vi "qc5psm3.vi"() -> ()   [LabVIEW 2020]
uses:
  <instrlib>/CAEN PSM/CAEN PSM.lvlib
panel:
  in  "Tab Control":enum32{"Page 1"}(tab)
  in  "Tab Control 3":enum32{"Page 1", "Page 2", "Page 3"}(tab)
  out "XY Graph":cluster{"X":dbl, "Y":dbl}[](graph)
  out "XY Graph 2":cluster{"X":dbl, "Y":dbl}[](graph)
  out "XY Graph 3":cluster{"Y":dbl[], "Y":dbl[]}[](graph)
  out "STATUS":string
  in  "Tab Control 2":enum32{"Page 1", "Page 2"}(tab)
  out "RDW":bool
  out "VMON":dbl(graph)
  out "IMON":dbl(graph)
  out "Shutting  DOWN":bool
  out "Vmon (Actual voltage level )":dbl
  out "Imon (Actual current level )":dbl
  out "OVC 2":bool
  out "OVV 2":bool
  out "COUNT VALUE":dynamicdata(graph)
  in  "count Time(sec)":dbl=60.0
  in  "Final Voltage":dbl=4900.0
  in  "V_step 1":dbl=200.0
  in  "VISA resource name":refnum<visa-resource-name>
  in  "Voltage ramp up (0 V/s)":u16 max=999
  in  "Voltage Max (0.0 V)":u16 max=9999
  in  "Board Address":i8 max=31
  in  "Vset_initial":dbl=200.0
  out "R calc":dbl
  in  "START AGAIN":bool
  out "Channel Status":T1(array[cluster])
  in  "Channel (0)":u8=1
  in  "Req (Mohm)":dbl
  in  "stop":bool
  in  "Middle Volt":dbl=3000.0
  in  "V step 2":dbl=100.0
  out "COUNT ON  TIMES":i16
  in  "device name (NI USB 6009)":tag="Dev1"
  out "Counts":dbl
  out "time eclapsed":i32
  out "I set status":dbl
  # "VOLTAGE RAMPUP SCHEME"
  # "INITIAL SETTING"
  # "RATE MEASUREMENT"
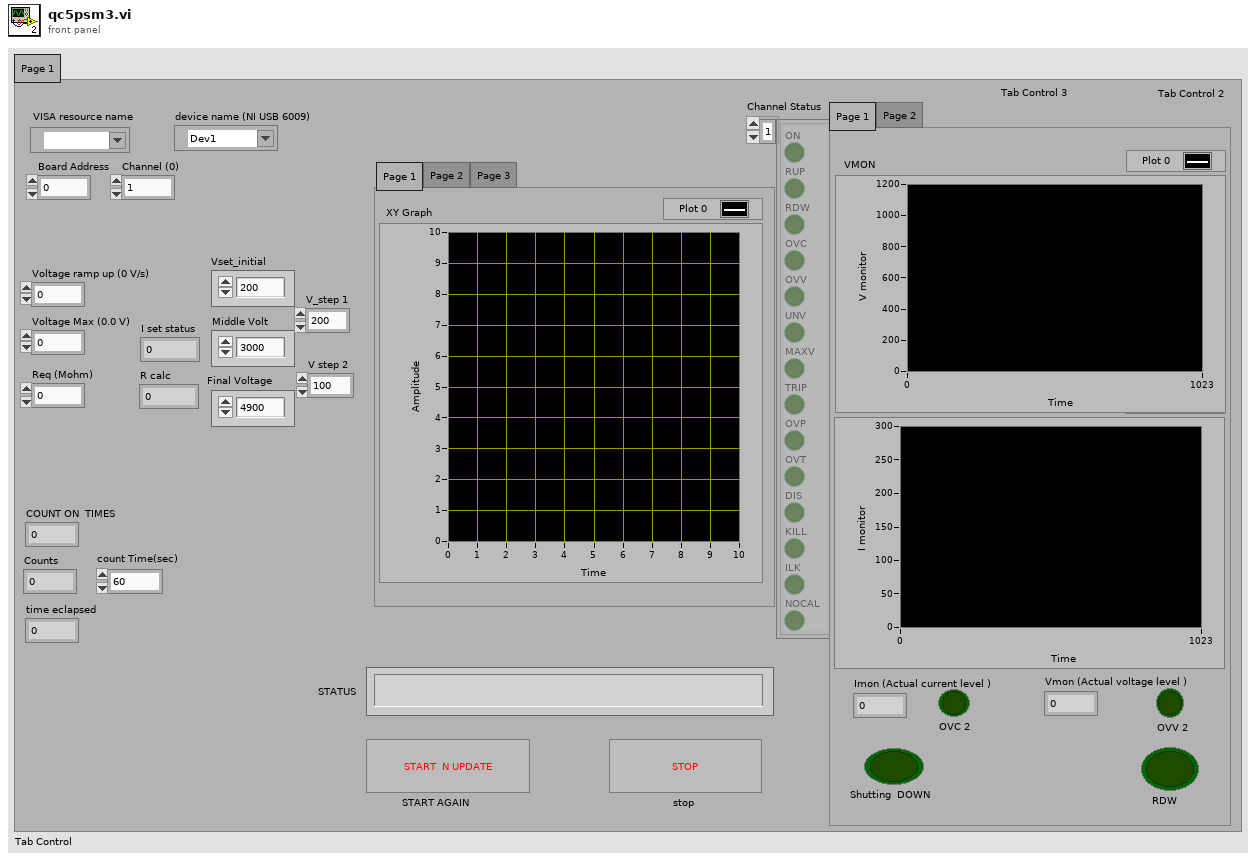
[diagram p1: front panel]
types:
  T1 = cluster{"ON":bool, "RUP":bool, "RDW":bool, "OVC":bool, "OVV":bool, "UNV":bool, "MAXV":bool, "TRIP":bool, "OVP":bool, "OVT":bool, "DIS":bool, "KILL":bool, "ILK":bool, "NOCAL":bool}[]
  T2 = cluster{"Baud Rate":u32, "Parity":enum16{"None", "Odd", "Even", "Mark", "Space"}, "Data Bits":u16, "Stop Bits":u16, "Flow Control":u16}
  T3 = typedef "CAEN PSM.lvlib/BoardHandle.ctl" = cluster{"VISA resource name":refnum<visa-resource-name>, "Board address":i8, "NChannels":u8}
  T4 = cluster{"ON":bool, "RUP":bool, "RDW":bool, "OVC":bool, "OVV":bool, "UNV":bool, "MAXV":bool, "TRIP":bool, "OVP":bool, "OVT":bool, "DIS":bool, "KILL":bool, "ILK":bool, "NOCAL":bool}
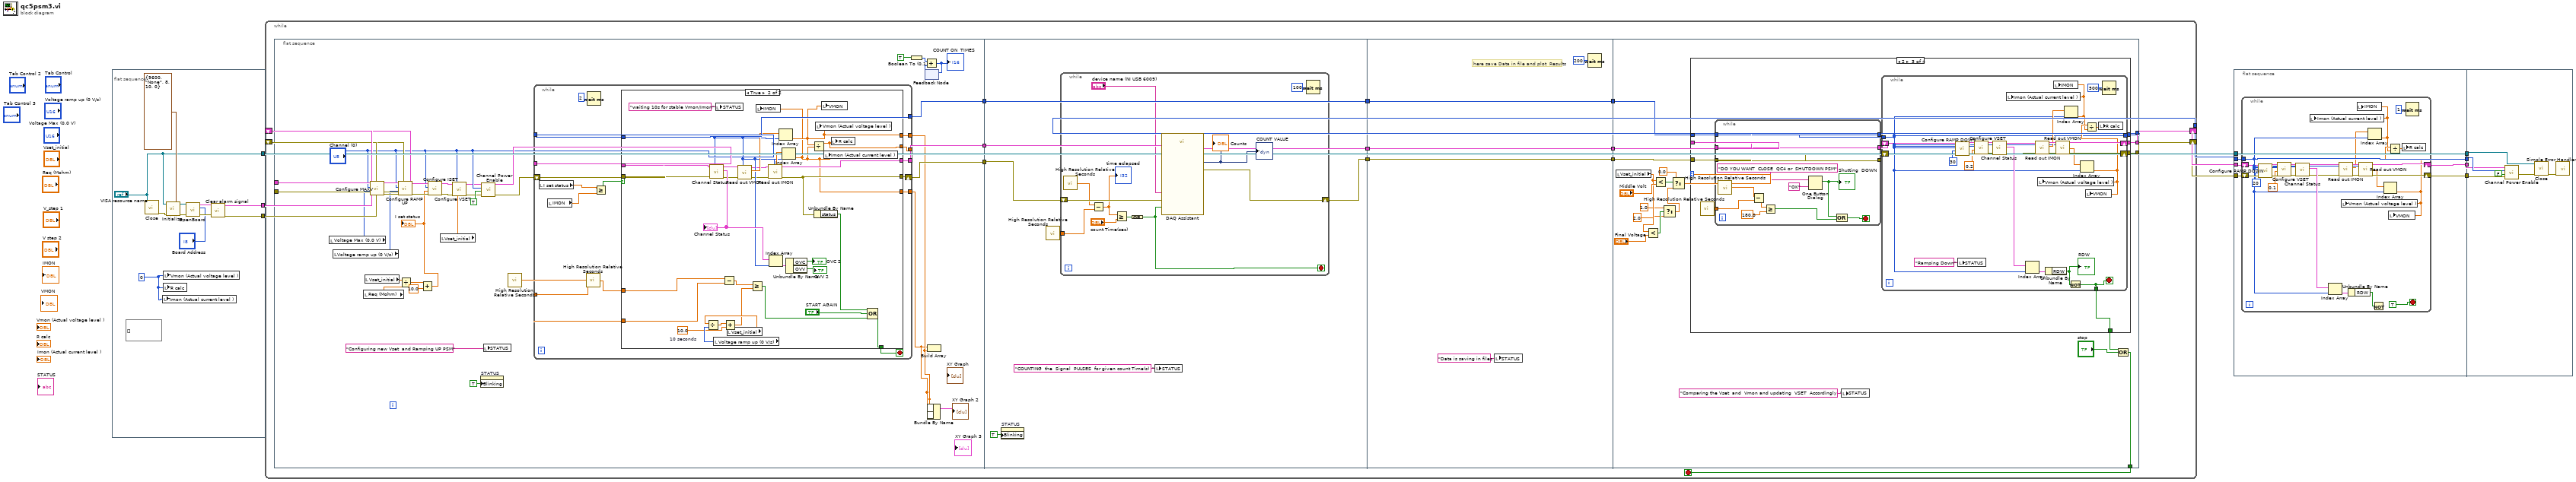
[diagram p0: block diagram]
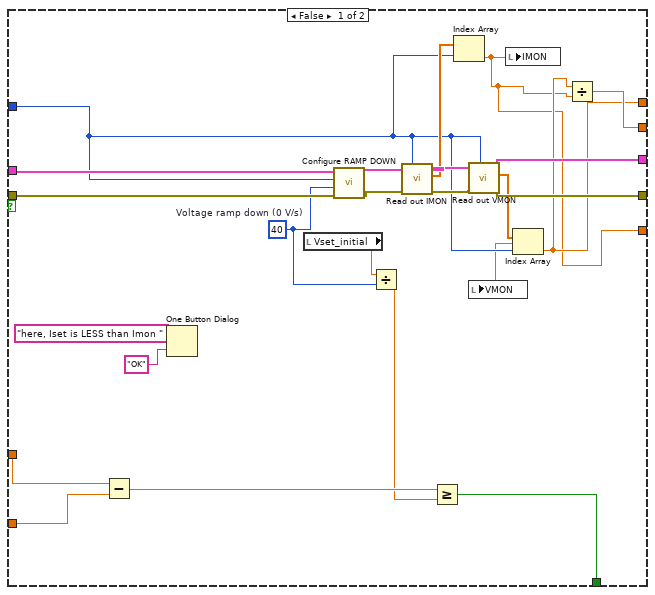
[diagram p2: hidden frame]
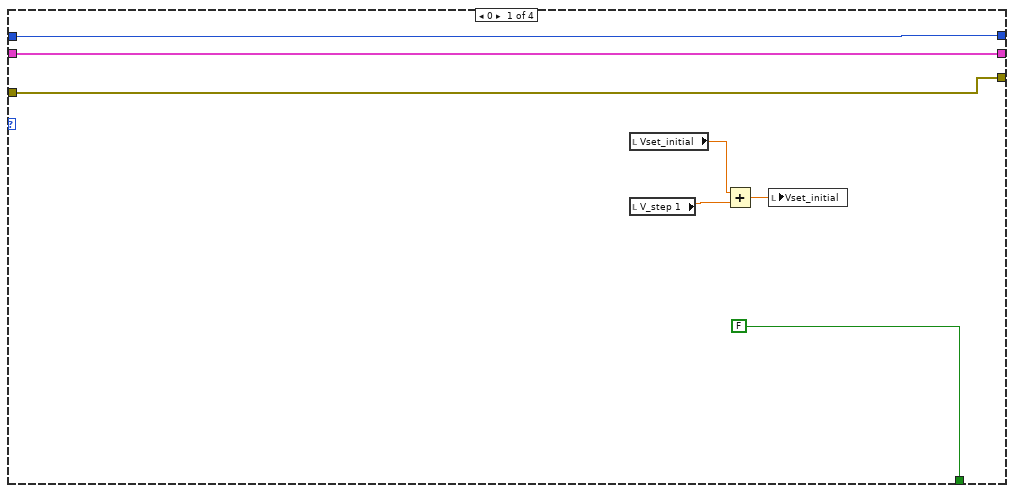
[diagram p3: hidden frame]
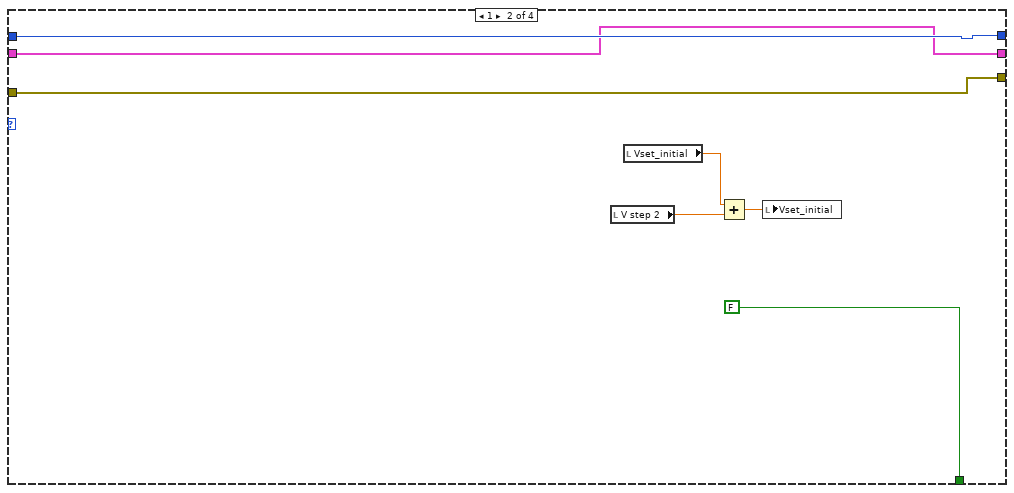
[diagram p4: hidden frame]
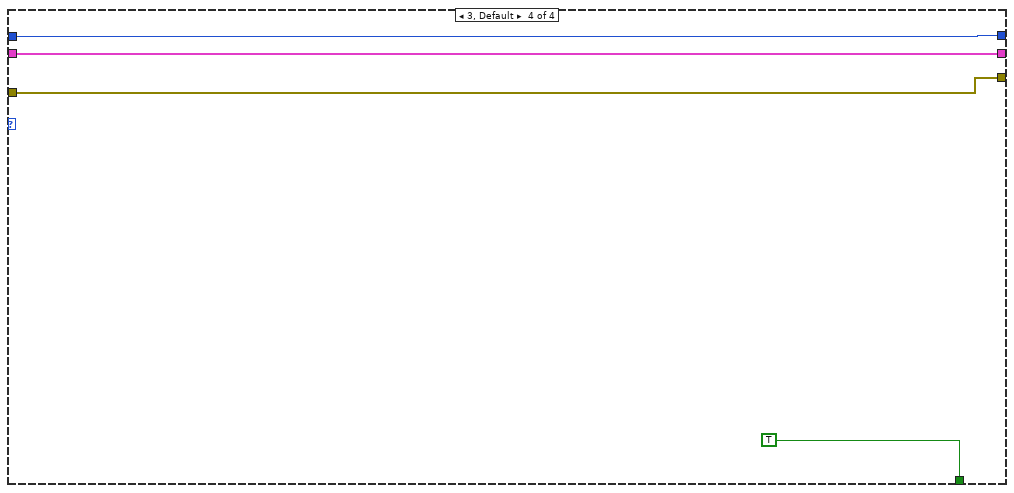
[diagram p5: hidden frame]
diagram:
  n1 = flat-sequence {
    tunnel: ["VISA resource name"] -> w10
    tunnel: [w15] -> w8
    tunnel: [w14] -> w7
    frame #0 {
      (unwired) void[][] []
      w11 = 0
      n2 = call <instrlib>:"Close.vi"("VISA resource name"="VISA resource name") -> ("error out"=w13:errorcluster)  [unwired: 10 in]
      n3 = local write "Imon (Actual current level )"(w11) -> ()
      n4 = local write "Vmon (Actual voltage level )"(w11) -> ()
      n5 = local write "R calc"(w11) -> ()
      n6 = call <instrlib>:"Initialize.vi"("Serial Configuration"=T2 {"Baud Rate"=9600, "Parity"=enum."None", "Data Bits"=8, "Stop Bits"=10, "Flow Control"=0}, "error in (no error)"=w13, "VISA resource name"="VISA resource name") -> ("error out"=w12:errorcluster, "VISA resource name out"=w20:refnum<visa-resource-name>)  [unwired: 7 in]
      n7 = call <instrlib>:"OpenBoard.vi"("error in (no error)"=w12, "Board Address"="Board Address", "VISA resource name"=w20) -> ("error out"=w18:errorcluster, "BoardHandle"=w19:T3)  [unwired: 7 in]
      n8 = call <instrlib>:"Clear alarm signal.vi"("error in (no error)"=w18, "BoardHandle"=w19) -> ("error out"=w14:errorcluster, "BoardHandle out"=w15:T3)  [unwired: 8 in]
    }
  }
  n9 = while {
    tunnel: [w36] -> w9
    shift-right: [w33] -> w6
    shift-left: w8 -> [w35]
    shift-right: [w28] -> w5
    shift-left: w7 -> [w34]
    stop <- w32 stop-if-true
    n10 = flat-sequence {
      tunnel: [w73] -> w31
      tunnel: [w52] -> w30
      tunnel: [w51] -> w29
      tunnel: w35 -> [w72]
      tunnel: w34 -> [w71]
      tunnel: w31 -> [w150]
      tunnel: [w150] -> w27
      tunnel: w30 -> [w149]
      tunnel: [w149] -> w25
      tunnel: w29 -> [w148]
      tunnel: [w147] -> w23
      tunnel: w27 -> [w166]
      tunnel: [w166] -> w26
      tunnel: w25 -> [w165]
      tunnel: [w165] -> w24
      tunnel: w23 -> [w164]
      tunnel: [w164] -> w22
      tunnel: [w169] -> w28
      tunnel: [w168] -> w33
      tunnel: [w172] -> w36
      tunnel: w26 -> [w173]
      tunnel: w24 -> [w171]
      tunnel: w22 -> [w170]
      tunnel: [w175] -> w32
      frame #0 {
        n11 = local read "Voltage Max (0.0 V)"() -> (w67:u16)
        n12 = local read "Voltage ramp up (0 V/s)"() -> (w66:u16)
        n13 = local read "Req (Mohm)"() -> (w56:dbl)
        n14 = local read "Vset_initial"() -> (w57:dbl)
        n15 = call <instrlib>:"Configure MAXV.vi"("error in (no error)"=w71, "Voltage Max (0.0 V)"=w67, "Channel (0)"="Channel (0)", "BoardHandle"=w72) -> ("error out"=w68:errorcluster, "BoardHandle out"=w69:T3)  [unwired: 6 in]
        n16 = call <instrlib>:"Configure RAMP UP.vi"("error in (no error)"=w68, "Voltage ramp up (0 V/s)"=w66, "Channel (0)"="Channel (0)", "BoardHandle"=w69) -> ("error out"=w62:errorcluster, "BoardHandle out"=w64:T3)  [unwired: 6 in]
        n17 = Divide(x=w57, y=w56) -> (x/y=w59:dbl)
        n18 = Add(x=w59, y=10.0) -> (x+y=w49:dbl)
        "I set status" <- w49
        n19 = call <instrlib>:"Configure ISET.vi"("error in (no error)"=w62, "Current Limit (0.00 uA)"=w49, "Channel (0)"="Channel (0)", "BoardHandle"=w64) -> ("error out"=w61:errorcluster, "BoardHandle out"=w63:T3)  [unwired: 6 in]
        n20 = local read "Vset_initial"() -> (w60:dbl)
        n21 = call <instrlib>:"Configure VSET.vi"("error in (no error)"=w61, "Voltage Level (0.0 V)"=w60, "Channel (0)"="Channel (0)", "BoardHandle"=w63) -> ("error out"=w54:errorcluster, "BoardHandle out"=w53:T3)  [unwired: 6 in]
        n22 = property on="STATUS" class="Str"("Blinking"=TRUE) -> ()  [unwired: 2 in, 2 out]
        n23 = call <instrlib>:"Channel Power Enable.vi"("error in (no error)"=w54, "Enable (OFF)"=TRUE, "Channel (0)"="Channel (0)", "BoardHandle"=w53) -> ("error out"=w70:errorcluster, "BoardHandle out"=w74:T3)  [unwired: 6 in]
        n24 = local write "STATUS"("Configuring new Vset  and Ramping UP PSM" ("STATUS")) -> ()
        n25 = call <vilib>:"High Resolution Relative Seconds.vi"() -> ("relative seconds"=w50:dbl)
        n26 = while {
          shift-right: [w85] -> w51
          shift-left: w70 -> [w86]
          tunnel: [w84] -> w52
          tunnel: [w89] -> w73
          tunnel: w74 -> [w87]
          tunnel: "Channel (0)" -> [w89]
          tunnel: w50 -> [w82]
          tunnel: [w77] -> w38
          tunnel: [w75] -> w42
          tunnel: [w76] -> w37
          stop <- w81 stop-if-true
          n27 = local read "I set status"() -> (w80:dbl)
          n28 = local read "IMON"() -> (w78:dbl)
          n29 = call <vilib>:"High Resolution Relative Seconds.vi"() -> ("relative seconds"=w79:dbl)
          n30 = Wait (ms)(milliseconds to wait=u32 2) -> ()  [unwired: 1 out]
          n31 = Greater Or Equal?(x=w80, y=w78) -> (x >= y?=w83:bool)
          n32 = case shown="True" w83 {
            tunnel: w89 -> [w96 w137]
            tunnel: w87 -> [w112 w136]
            tunnel: w86 -> [w111 w135]
            tunnel: [w99 w134] -> w85
            tunnel: [w100 w133] -> w84
            tunnel: w82 -> [w110 w128]
            tunnel: [w105 w123] -> w81
            tunnel: w79 -> [w93 w117]
            tunnel: [w91 w115] -> w77
            tunnel: [w90 w114] -> w76
            tunnel: [w92 w113] -> w75
            frame False {
              w107 = u16 40  # Voltage ramp down (0 V/s)
              n33 = Subtract(x=w93, y=w110) -> (x-y=w109:dbl)
              n34 = One Button Dialog(message="here, Iset is LESS than Imon ", button name ("OK")="OK") -> ()  [unwired: 1 out]
              n35 = local read "Vset_initial"() -> (w108:dbl)
              n36 = call <instrlib>:"Configure RAMP DOWN.vi"("error in (no error)"=w111, "Voltage ramp down (0 V/s)"=w107, "Channel (0)"=w96, "BoardHandle"=w112) -> ("error out"=w103:errorcluster, "BoardHandle out"=w104:T3)  [unwired: 6 in]
              n37 = Divide(x=w108, y=w107) -> (x/y=w106:dbl)
              n38 = call <instrlib>:"Read out IMON.vi"("Channel"=w96, "error in (no error)"=w103, "BoardHandle"=w104) -> ("error out"=w101:errorcluster, "IMon values (uA)"=w98:dbl[], "BoardHandle out"=w102:T3)  [unwired: 5 in, 1 out]
              n39 = Greater Or Equal?(x=w109, y=w106) -> (x >= y?=w105:bool)
              n40 = Index Array(array=w98, index=w96) -> (element=w90:dbl)
              n41 = call <instrlib>:"Read out VMON.vi"("Channel"=w96, "error in (no error)"=w101, "BoardHandle"=w102) -> ("error out"=w99:errorcluster, "VMon values (V)"=w97:dbl[], "BoardHandle out"=w100:T3)  [unwired: 6 in]
              n42 = local write "IMON"(w90) -> ()
              n43 = Index Array(array=w97, index=w96) -> (element=w91:dbl)
              n44 = local write "VMON"(w91) -> ()
              n45 = Divide(x=w91, y=w90) -> (x/y=w92:dbl)
            }
            frame True {
              w119 = 10.0  # 10 seconds
              n46 = call <instrlib>:"Channel Status.vi"("Channel"=w137, "error in (no error)"=w135, "BoardHandle"=w136) -> ("error out"=w131:errorcluster, "Channel Status Array"=w142:T1, "BoardHandle out"=w132:T3)  [unwired: 5 in, 1 out]
              "Channel Status" <- w142
              n47 = local read "Voltage ramp up (0 V/s)"() -> (w121:u16)
              n48 = local write "STATUS"("waiting 10s for stable Vmon/Imon" ("STATUS")) -> ()
              n49 = Subtract(x=w117, y=w128) -> (x-y=w125:dbl)
              n50 = local read "Vset_initial"() -> (w122:dbl)
              n51 = Divide(x=w122, y=w121) -> (x/y=w120:dbl)
              n52 = Add(x=w120, y=w119) -> (x+y=w118:dbl)
              n53 = call <instrlib>:"Read out VMON.vi"("Channel"=w137, "error in (no error)"=w131, "BoardHandle"=w132) -> ("error out"=w129:errorcluster, "VMon values (V)"=w143:dbl[], "BoardHandle out"=w130:T3)  [unwired: 6 in]
              n54 = Greater Or Equal?(x=w125, y=w118) -> (x >= y?=w127:bool)
              n55 = call <instrlib>:"Read out IMON.vi"("Channel"=w137, "error in (no error)"=w129, "BoardHandle"=w130) -> ("error out"=w134:errorcluster, "IMon values (uA)"=w138:dbl[], "BoardHandle out"=w133:T3)  [unwired: 5 in, 1 out]
              n56 = Index Array(array=w142, index=w137) -> (element=w141:T4)
              n57 = Index Array(array=w143, index=w137) -> (element=w115:dbl)
              n58 = Index Array(array=w138, index=w137) -> (element=w114:dbl)
              n59 = local write "IMON"(w114) -> ()
              n60 = Unbundle By Name(w141) -> ("OVC"=→"OVC 2":bool, "OVV"=→"OVV 2":bool)
              n61 = Divide(x=w115, y=w114) -> (x/y=w113:dbl)
              n62 = Unbundle By Name(w134) -> ("status"=w124:bool)
              n63 = local write "Vmon (Actual voltage level )"(w115) -> ()
              n64 = local write "VMON"(w115) -> ()
              n65 = local write "Imon (Actual current level )"(w114) -> ()
              n66 = local write "R calc"(w113) -> ()
              n67 = Compound Arithmetic op=OR(w124, "START AGAIN", w127) -> (w123:bool)
            }
          }
        }
        n68 = Boolean To (0,1)(Boolean=TRUE) -> (0, 1=w46:i16)
        n69 = feedback #1() -> (w48:i16)  [unwired: 1 in]
        n70 = Add(x=w46, y=w48) -> (x+y=w47:i16)
        "COUNT ON  TIMES" <- w47
        n71 = feedback-in #1(w47) -> ()
        n72 = Build Array(w37, w38) -> (w40:dbl[])
        n73 = Bundle By Name(w38, w37) -> (→"XY Graph 2":cluster{})  [unwired: 1 in]
      }
      frame #1 {
        n74 = property on="STATUS" class="Str"("Blinking"=TRUE) -> ()  [unwired: 2 in, 2 out]
        n75 = call <vilib>:"High Resolution Relative Seconds.vi"() -> ("relative seconds"=w146:dbl)
        n76 = while {
          shift-right: [w160] -> w147
          shift-left: w148 -> [w161]
          tunnel: w146 -> [w155]
          stop <- w152 stop-if-true
          n77 = call <vilib>:"High Resolution Relative Seconds.vi"() -> ("relative seconds"=w157:dbl)
          n78 = Subtract(x=w157, y=w155) -> (x-y=w158:dbl)
          "time eclapsed" <- w158
          n79 = Greater Or Equal?(x=w158, y="count Time(sec)") -> (x >= y?=w156:bool)
          n80 = Compound Arithmetic op=OR(w156) -> (w152:bool)
          n81 = call "DAQ Assistant"("error in"=w161, "stop (F)"=w152, "device name"="device name (NI USB 6009)") -> ("data"=→"Counts" →"COUNT VALUE":dynamicdata, "error out"=w160:errorcluster)  [unwired: 13 in, 2 out]
          n82 = Wait (ms)(milliseconds to wait=u32 100) -> ()  [unwired: 1 out]
        }
        n83 = local write "STATUS"("COUNTING  the  Signal  PULSES  for given count Time(s)  " ("STATUS")) -> ()
      }
      frame #2 {
        # "here save Data in file and plot  Results"
        n84 = local write "STATUS"("Data is saving in files " ("STATUS")) -> ()
        n85 = Wait (ms)(milliseconds to wait=u32 200) -> ()  [unwired: 1 out]
      }
      frame #3 {
        n86 = local read "Vset_initial"() -> (w180:dbl)
        n87 = Less?(x=w180, y="Final Voltage") -> (x < y?=w183:bool)
        n88 = Less?(x=w180, y="Middle Volt") -> (x < y?=w185:bool)
        n89 = Select(t=1.0, s=w183, f=2.0) -> (s? t:f=w181:dbl)
        n90 = Select(t=0.0, s=w185, f=w181) -> (s? t:f=w186:dbl)
        n91 = case shown="2" w186 {
          tunnel: [FALSE FALSE w208 TRUE] -> w174
          tunnel: w173 -> [w189 w196 w203 w251]
          tunnel: [w189 w196 w211 w251] -> w172
          tunnel: w171 -> [w188 w195 w205 w250]
          tunnel: w170 -> [w187 w194 w207 w249]
          tunnel: [w187 w194 w209 w249] -> w169
          tunnel: [w188 w195 w210 w250] -> w168
          frame 0 {
            n92 = local read "Vset_initial"() -> (w193:dbl)
            n93 = local read "V_step 1"() -> (w191:dbl)
            n94 = Add(x=w193, y=w191) -> (x+y=w192:dbl)
            n95 = local write "Vset_initial"(w192) -> ()
          }
          frame 1 {
            n96 = local read "V step 2"() -> (w198:dbl)
            n97 = local read "Vset_initial"() -> (w200:dbl)
            n98 = Add(x=w200, y=w198) -> (x+y=w199:dbl)
            n99 = local write "Vset_initial"(w199) -> ()
          }
          frame 2 {
            n100 = call <vilib>:"High Resolution Relative Seconds.vi"() -> ("relative seconds"=w201:dbl)
            n101 = while {
              tunnel: w207 -> [w223]
              tunnel: [w223] -> w206
              tunnel: w205 -> [w222]
              tunnel: [w222] -> w204
              tunnel: w203 -> [w221]
              tunnel: [w221] -> w202
              tunnel: w201 -> [w217]
              stop <- w213 stop-if-true
              n102 = call <vilib>:"High Resolution Relative Seconds.vi"() -> ("relative seconds"=w218:dbl)
              n103 = Subtract(x=w218, y=w217) -> (x-y=w216:dbl)
              n104 = Greater Or Equal?(x=w216, y=180.0) -> (x >= y?=w214:bool)
              n105 = One Button Dialog(message="DO YOU WANT  CLOSE  QC4 or  SHUTDOWN PSM", button name ("OK")="OK") -> (true=w212:bool)
              "Shutting  DOWN" <- w212
              n106 = Compound Arithmetic op=OR(w212, w214) -> (w213:bool)
            }
            n107 = while {
              tunnel: w202 -> [w226]
              shift-right: [w246] -> w210
              shift-left: w204 -> [w248]
              shift-right: [w245] -> w209
              shift-left: w206 -> [w247]
              tunnel: [w226] -> w211
              tunnel: [w225] -> w208
              stop <- w225 stop-if-true
              n108 = call <instrlib>:"Configure RAMP DOWN.vi"("error in (no error)"=w247, "Voltage ramp down (0 V/s)"=u16 30, "Channel (0)"=w226, "BoardHandle"=w248) -> ("error out"=w241:errorcluster, "BoardHandle out"=w242:T3)  [unwired: 6 in]
              n109 = local write "STATUS"("Ramping Down" ("STATUS")) -> ()
              n110 = call <instrlib>:"Configure VSET.vi"("error in (no error)"=w241, "Voltage Level (0.0 V)"=0.2, "Channel (0)"=w226, "BoardHandle"=w242) -> ("error out"=w238:errorcluster, "BoardHandle out"=w239:T3)  [unwired: 6 in]
              n111 = call <instrlib>:"Channel Status.vi"("Channel"=w226, "error in (no error)"=w238, "BoardHandle"=w239) -> ("error out"=w233:errorcluster, "Channel Status Array"=w237:T1, "BoardHandle out"=w232:T3)  [unwired: 5 in, 1 out]
              n112 = Index Array(array=w237, index=w226) -> (element=w236:T4)
              n113 = call <instrlib>:"Read out IMON.vi"("Channel"=w226, "BoardHandle"=w232) -> ("IMon values (uA)"=w230:dbl[], "BoardHandle out"=w231:T3)  [unwired: 6 in, 2 out]
              n114 = Unbundle By Name(w236) -> ("RDW"=w235:bool)
              "RDW" <- w235
              n115 = call <instrlib>:"Read out VMON.vi"("Channel"=w226, "error in (no error)"=w233, "BoardHandle"=w231) -> ("error out"=w245:errorcluster, "VMon values (V)"=w243:dbl[], "BoardHandle out"=w246:T3)  [unwired: 6 in]
              n116 = Index Array(array=w230, index=w226) -> (element=w227:dbl)
              n117 = local write "Imon (Actual current level )"(w227) -> ()
              n118 = local write "IMON"(w227) -> ()
              n119 = Not(x=w235) -> (.not. x?=w225:bool)
              n120 = Index Array(array=w243, index=w226) -> (element=w228:dbl)
              n121 = local write "Vmon (Actual voltage level )"(w228) -> ()
              n122 = Divide(x=w228, y=w227) -> (x/y=w229:dbl)
              n123 = local write "VMON"(w228) -> ()
              n124 = local write "R calc"(w229) -> ()
              n125 = Wait (ms)(milliseconds to wait=u32 500) -> ()  [unwired: 1 out]
            }
          }
          frame 3, Default {
          }
        }
        n126 = local write "STATUS"("Comparing the Vset  and  Vmon and updating  VSET  Accordingly  " ("STATUS")) -> ()
        n127 = Compound Arithmetic op=OR(w174, "stop") -> (w175:bool)
      }
    }
  }
  n128 = flat-sequence {
    tunnel: w5 -> [w256]
    tunnel: w6 -> [w257]
    tunnel: w9 -> [w253]
    tunnel: w10 -> [w258]
    tunnel: [w258] -> w4
    tunnel: [w253] -> w3
    tunnel: [w255] -> w2
    tunnel: [w254] -> w1
    tunnel: w4 -> [w287]
    tunnel: w3 -> [w285]
    tunnel: w2 -> [w284]
    tunnel: w1 -> [w283]
    frame #0 {
      n129 = while {
        tunnel: w253 -> [w270]
        shift-right: [w280] -> w255
        shift-left: w257 -> [w282]
        shift-right: [w279] -> w254
        shift-left: w256 -> [w281]
        stop <- TRUE stop-if-true
        n130 = call <instrlib>:"Configure RAMP DOWN.vi"("error in (no error)"=w281, "Voltage ramp down (0 V/s)"=u16 20, "Channel (0)"=w270, "BoardHandle"=w282) -> ("error out"=w275:errorcluster, "BoardHandle out"=w276:T3)  [unwired: 6 in]
        n131 = call <instrlib>:"Configure VSET.vi"("error in (no error)"=w275, "Voltage Level (0.0 V)"=0.1, "Channel (0)"=w270, "BoardHandle"=w276) -> ("error out"=w272:errorcluster, "BoardHandle out"=w273:T3)  [unwired: 6 in]
        n132 = call <instrlib>:"Channel Status.vi"("Channel"=w270, "error in (no error)"=w272, "BoardHandle"=w273) -> ("error out"=w266:errorcluster, "Channel Status Array"=w271:T1, "BoardHandle out"=w265:T3)  [unwired: 5 in, 1 out]
        n133 = Index Array(array=w271, index=w270) -> (element=w269:T4)
        n134 = call <instrlib>:"Read out IMON.vi"("Channel"=w270, "BoardHandle"=w265) -> ("IMon values (uA)"=w263:dbl[], "BoardHandle out"=w264:T3)  [unwired: 6 in, 2 out]
        n135 = Unbundle By Name(w269) -> ("RDW"=w268:bool)
        n136 = call <instrlib>:"Read out VMON.vi"("Channel"=w270, "error in (no error)"=w266, "BoardHandle"=w264) -> ("error out"=w279:errorcluster, "VMon values (V)"=w277:dbl[], "BoardHandle out"=w280:T3)  [unwired: 6 in]
        n137 = Index Array(array=w263, index=w270) -> (element=w260:dbl)
        n138 = local write "Imon (Actual current level )"(w260) -> ()
        n139 = local write "IMON"(w260) -> ()
        n140 = Not(x=w268) -> ()  [unwired: 1 out]
        n141 = Index Array(array=w277, index=w270) -> (element=w261:dbl)
        n142 = local write "Vmon (Actual voltage level )"(w261) -> ()
        n143 = Divide(x=w261, y=w260) -> (x/y=w262:dbl)
        n144 = local write "VMON"(w261) -> ()
        n145 = local write "R calc"(w262) -> ()
        n146 = Wait (ms)(milliseconds to wait=u32 1) -> ()  [unwired: 1 out]
      }
    }
    frame #1 {
      n147 = call <instrlib>:"Channel Power Enable.vi"("error in (no error)"=w283, "Enable (OFF)"=FALSE, "Channel (0)"=w285, "BoardHandle"=w284) -> ("error out"=w289:errorcluster)  [unwired: 6 in, 1 out]
      n148 = call <instrlib>:"Close.vi"("error in (no error)"=w289, "VISA resource name"=w287) -> ("error out"=w288:errorcluster)  [unwired: 9 in]
      n149 = call <vilib>:"Simple Error Handler.vi"("error in (no error)"=w288) -> ()  [unwired: 4 in, 5 out]
    }
  }
